vi "EndOfPathHandler.vi"(8 "MaxAccel":dbl, 9 "MaxVel":dbl, 10 "RobotLocation":cluster{dbl, dbl}, 11 "Path":cluster{"x":dbl, "y":dbl}[](array[cluster])=[{"x"=0.0, "y"=10.0}, {"x"=0.0, "y"=80.0}, {"x"=85.0, "y"=140.0}, {"x"=85.0, "y"=20.0}, {"x"=40.0, "y"=15.0}]) -> (0 "Done":bool, 1 "Override":bool, 2 "ExtraPowerOut":dbl, 3 "VelOut":dbl)   [LabVIEW 2016]
uses:
  <vilib>/addons/control/pid/pid.llb/PID (DBL).vi
  <vilib>/addons/control/pid/NI_PID_pid.lvlib
panel:
  in  "PID gains":T1 {"derivative time (Td, min)" format="%.3f"; "integral time (Ti, min)" format="%.3f"; "proportional gain (Kc)" format="%.3f"}
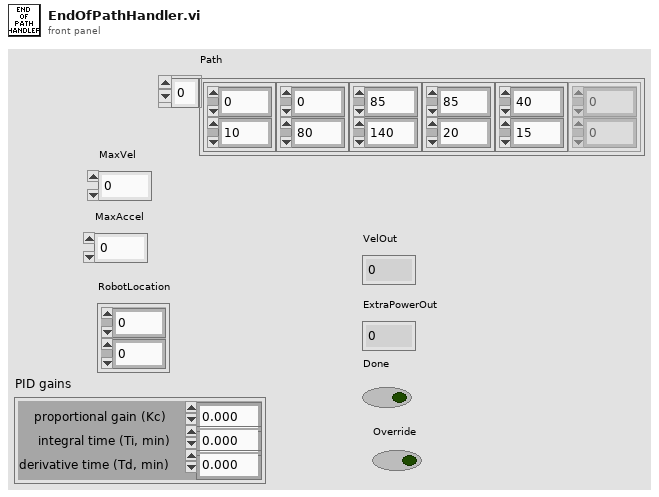
[diagram p1: front panel]
types:
  T1 = cluster{"proportional gain (Kc)":dbl, "integral time (Ti, min)":dbl, "derivative time (Td, min)":dbl}
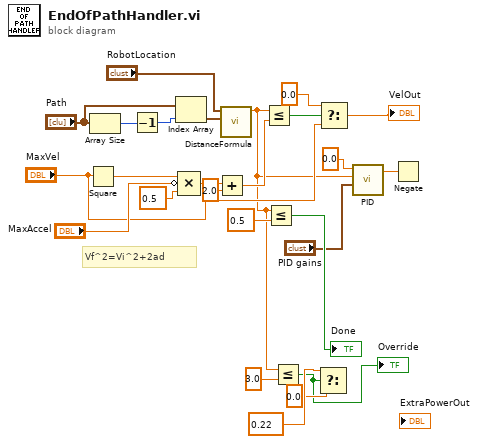
[diagram p0: block diagram]
diagram:
  # "Vf^2=Vi^2+2ad"
  n1 = Square(x="MaxVel") -> (x^2=w9:dbl)
  n2 = Array Size(array="Path") -> (size(s)=w23:i32)
  n3 = Decrement(x=w23) -> (x-1=w22:i32)
  n4 = Index Array(array="Path", index=w22) -> (element=w20:cluster{"x":dbl, "y":dbl})
  n5 = Compound Arithmetic op=MULTIPLY(w9, invert "MaxAccel", 0.5 ("value")) -> (w8:dbl)
  n6 = Add(x=w8, y=2.0) -> (x+y=w7:dbl)
  n7 = call "DistanceFormula.vi"("Point 2"=w20, "Point 1"="RobotLocation") -> ("Distance"=w4:dbl)  [unwired: 9 in]
  n8 = Less Or Equal?(x=w4, y=w7) -> (x <= y?=w16:bool)
  n9 = Less Or Equal?(x=w4, y=0.5) -> (x <= y?=→"Done":bool)
  n10 = Less Or Equal?(x=w4, y=3.0) -> (x <= y?=w1:bool)
  "Override" <- w1
  n11 = Select(t=0.22 ("ExtraPowerOut"), s=w1, f=0.0) -> ()  [unwired: 1 out]
  n12 = Select(t=0.0, s=w16, f="MaxVel") -> (s? t:f=→"VelOut":dbl)
  n13 = call-poly <vilib>:"PID.vi"("PID gains"="PID gains", "process variable"=w4, "setpoint"=0.0) -> ("output"=w10:dbl)  [unwired: 7 in, 1 out]
  n14 = Negate(x=w10) -> ()  [unwired: 1 out]
